vi "Create Temp ini.vi"(8 "error in":errorcluster, 11 "Original ini path":path=path "C:/Users/Tyler Doodeman/Desktop/Test/RTCtrlr.ini") -> (0 "error out":errorcluster, 3 "Temp ini path":path)   [LabVIEW 2015]
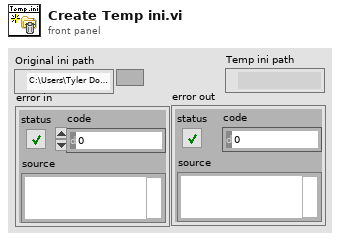
[diagram p1: front panel]
types:
  T1 = enum16{"open", "replace", "create", "open or create", "replace or create", "replace or create with confirmation"}
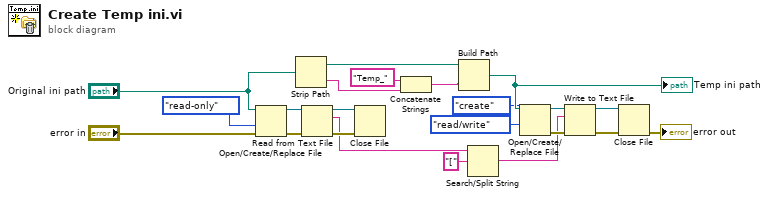
[diagram p0: block diagram]
diagram:
  n1 = Open/Create/Replace File(file path (use dialog)="Original ini path", error in="error in", access (0:read/write)=enum16{"read/write", "read-only", "write-only"}."read-only") -> (refnum out=w22:refnum<file>, error out=w21:errorcluster)  [unwired: 3 in, 1 out]
  n2 = Strip Path(path="Original ini path") -> (stripped path=w9:path, name=w5:string)
  n3 = Read from Text File(file (use dialog)=w22, error in=w21) -> (refnum out=w20:refnum<file>, text=w18:string, error out=w19:errorcluster)  [unwired: 2 in, 1 out]
  n4 = Close File(refnum=w20, error in=w19) -> ()  [unwired: 2 out]
  n5 = Concatenate Strings("Temp_" ("string"), w5) -> (w8:string)
  n6 = Build Path(base path=w9, name or relative path=w8) -> (appended path=w7:path)
  "Temp ini path" <- w7
  n7 = Search/Split String(string=w18, search string/char (-)="[") -> (match + rest of string=w12:string)  [unwired: 1 in, 2 out]
  n8 = Open/Create/Replace File(file path (use dialog)=w7, operation (0:open)=T1."create", access (0:read/write)=enum16{"read/write", "read-only", "write-only"}."read/write") -> (refnum out=w14:refnum<file>, error out=w13:errorcluster)  [unwired: 3 in, 1 out]
  n9 = Write to Text File(file (use dialog)=w14, text=w12, error in=w13) -> (refnum out=w1:refnum<file>, error out=w4:errorcluster)  [unwired: 1 in, 1 out]
  n10 = Close File(refnum=w1, error in=w4) -> (error out=→"error out":errorcluster)  [unwired: 1 out]
